vi "Normalizer.vi"(7 "Dataset_Stats":T1={"means"={"R"=0.5385, "G"=0.5348, "B"=0.551}, "stds"={"R"=0.3673, "G"=0.3673, "B"=0.3505}} {"stds"."R" format="%#_3g"; "stds"."G" format="%#_3g"; "stds"."B" format="%#_3g"; "means"."R" format="%#_3g"; "means"."G" format="%#_3g"; "means"."B" format="%#_3g"}, 9 "B":sgl[][](array[numeric]), 10 "G":sgl[][](array[numeric]), 11 "R":sgl[][](array[numeric])) -> (3 "Norm_Img_Out":sgl[][][](array[numeric]))   [LabVIEW 2024]
uses:
  <vilib>/Ngene/DeepLTK Anomaly Detection Addon/DeepLTK_Anomaly_Detection_Addon/API/Controls/NNPC_DS_Stats.ctl
  <vilib>/Ngene/DeepLTK Anomaly Detection Addon/DeepLTK_Anomaly_Detection_Addon/API/Controls/Image_Stats_RGB.ctl
  <vilib>/Ngene/DeepLTK Anomaly Detection Addon/DeepLTK_Anomaly_Detection_Addon/DeepLTK_Anomaly_Detection_Addon.lvlib
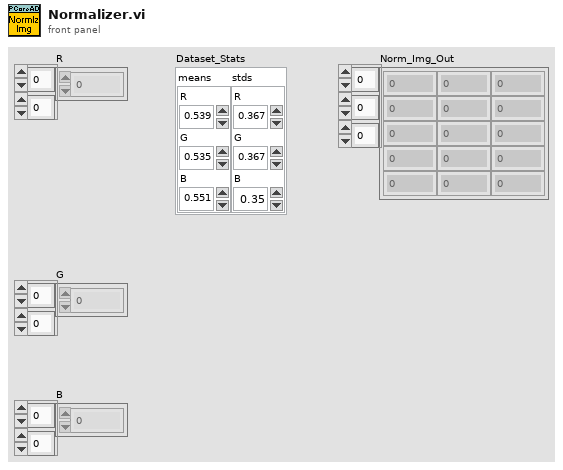
[diagram p1: front panel]
types:
  T1 = typedef "DeepLTK_Anomaly_Detection_Addon.lvlib/NNPC_DS_Stats.ctl" = cluster{"means":T2, "stds":T2}
  T2 = typedef "DeepLTK_Anomaly_Detection_Addon.lvlib/Image_Stats_RGB.ctl" = cluster{"R":sgl, "G":sgl, "B":sgl}
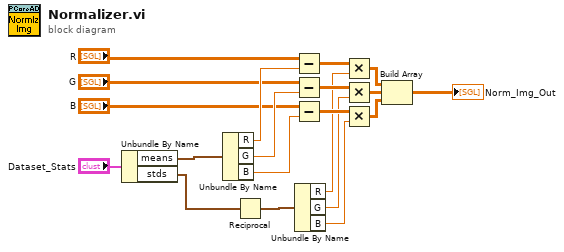
[diagram p0: block diagram]
diagram:
  n1 = Unbundle By Name("Dataset_Stats") -> ("means"=w7:T2, "stds"=w6:T2)
  n2 = Unbundle By Name(w7) -> ("R"=w13:sgl, "G"=w12:sgl, "B"=w11:sgl)
  n3 = Reciprocal(x=w6) -> (1/x=w5:T2)
  n4 = Subtract(x="R", y=w13) -> (x-y=w20:sgl[][])
  n5 = Subtract(x="G", y=w12) -> (x-y=w19:sgl[][])
  n6 = Subtract(x="B", y=w11) -> (x-y=w18:sgl[][])
  n7 = Unbundle By Name(w5) -> ("R"=w10:sgl, "G"=w9:sgl, "B"=w8:sgl)
  n8 = Multiply(x=w20, y=w10) -> (x*y=w17:sgl[][])
  n9 = Multiply(x=w19, y=w9) -> (x*y=w16:sgl[][])
  n10 = Multiply(x=w18, y=w8) -> (x*y=w15:sgl[][])
  n11 = Build Array(w17, w16, w15) -> (→"Norm_Img_Out":sgl[][][])
